vi "Vibration.vi"() -> ()   [LabVIEW 2012]
uses:
  <vilib>/Analysis/NI_AALPro.lvlib
panel:
  out "选项卡":T1(tab)
  in  "装置IP":string
  in  "?":bool
  in  "采样率(ksps)":T2(ring)=enum."105.468"
  in  "?":bool
  in  "?":bool
  in  "开始":bool
  in  "?":bool
  in  "设置装置网关":string
  in  "设置装置子网掩码":string
  in  "设置装置IP":string
  in  "?":bool
  in  "是否开启电流源":u8(knob)=1 scale=0.0..1.0
  in  "是否进行自校准":u8(knob) scale=0.0..1.0
  in  "?":bool
  in  "?":path
  in  "是否保存数据":u8(knob) scale=0.0..1.0
  in  "?":bool
  out "进度条":dbl(slide) scale=0.0..99.0
  out "字符串":string
  out "波形卡":enum32{"波形卡 1", "波形卡 2", "波形卡 3"}(tab)
  in  "AC/DC":bool
  in  "Y轴调整":dbl(knob)=5.0 min=0.0001 max=5.0 step=0.001 scale=0.0001..5.0
  out "?":dbl[][](graph)
  out "?":dbl[][](graph)
  in  "X轴调整":u32(knob)=50000 min=1000 max=50000 step=100 scale=1100.0..50000.0
  in  "通道1":bool=TRUE
  in  "通道2":bool=TRUE
  in  "通道3":bool=TRUE
  in  "通道4":bool=TRUE
  in  "灵敏度1(mv/g)":i32=1 min=1
  in  "灵敏度2(mv/g)":i32=1 min=1
  in  "灵敏度3(mv/g)":i32=1 min=1
  in  "灵敏度4(mv/g)":i32=1 min=1
  out "?":u16[](graph)
  out "转 \n速":u16(knob) scale=0.0..20000.0
  # "PageUp\nPageDown\n微调"
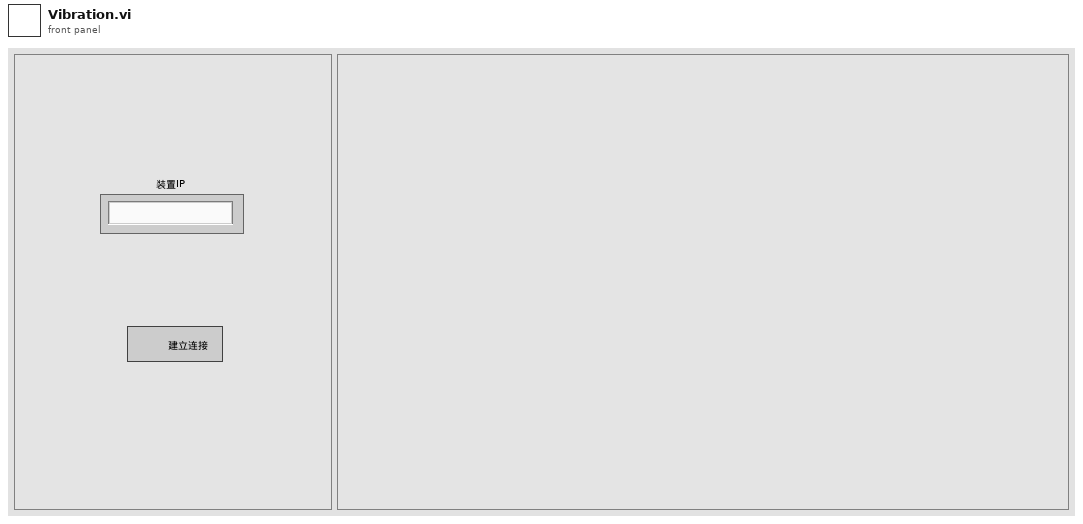
[diagram p1: front panel]
types:
  T1 = enum32{"选项卡 1", "选项卡 2", "选项卡 3", "选项卡 4", "选项卡 5", "选项卡 6", "选项卡 7"}
  T2 = enum16{"", "105.468", "52.734", "35.156", "26.367", "21.094", "17.578", "15.067", "13.184", "11.719", "10.545"}
  T3 = enum8{"Enabled", "Disabled", "Disabled and Grayed Out"}
  T4 = cluster{"refnum":refnum<file>, "refnum":refnum<file>, "refnum":refnum<file>, "refnum":refnum<file>, "refnum":refnum<file>, "SavePath":path, "SAVE?":bool, "connection ID":refnum<k5>}
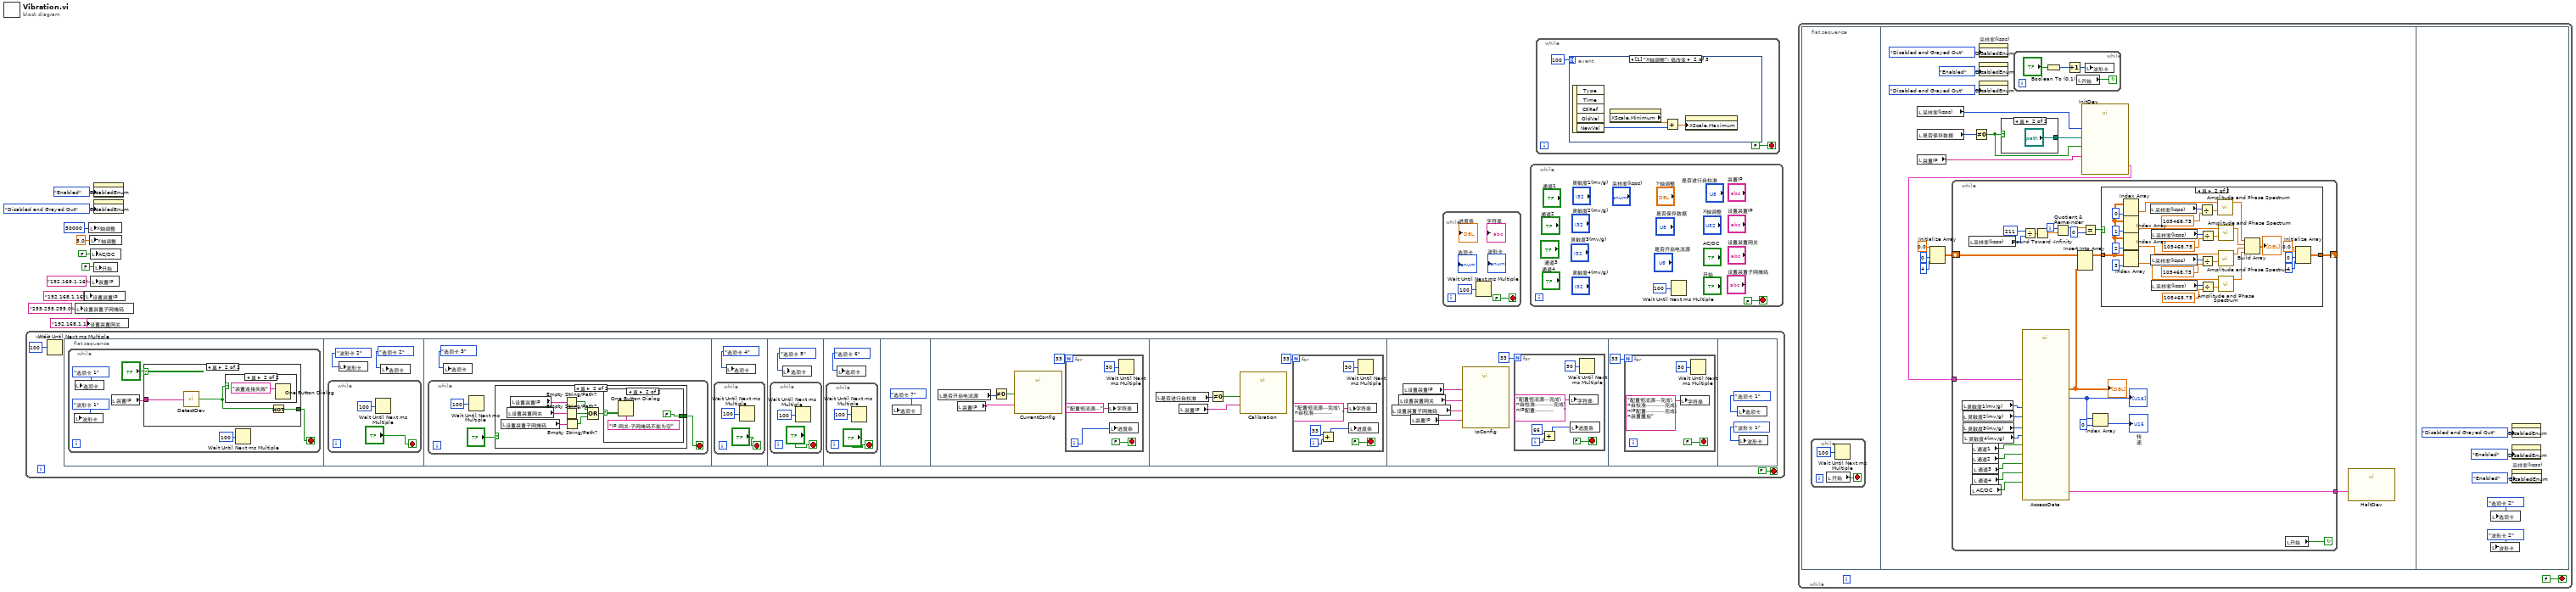
[diagram p0: block diagram]
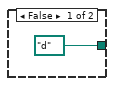
[diagram p3: hidden frame]
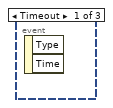
[diagram p4: hidden frame]
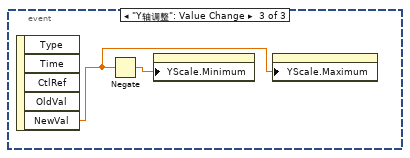
[diagram p5: hidden frame]
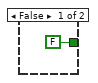
[diagram p6: hidden frame]
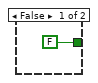
[diagram p8: hidden frame]
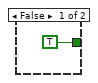
[diagram p9: hidden frame]
diagram:
  n1 = while {
    stop <- FALSE stop-if-true
    n2 = Wait Until Next ms Multiple(millisecond multiple=u32 100 ("毫秒倍数")) -> ()  [unwired: 1 out]
    n3 = flat-sequence {
      frame #0 {
        n4 = while {
          stop <- w17 stop-if-true
          n5 = local write "波形卡"(enum32{"波形卡 1", "波形卡 2", "波形卡 3"}."波形卡 1" ("波形卡")) -> ()
          n6 = local write "选项卡"(T1."选项卡 1" ("选项卡")) -> ()
          n7 = local read "装置IP"() -> (w13:string)
          n8 = case shown="真" "?" {
            tunnel: [FALSE w22] -> w17
            tunnel: w13 -> [_ w20]
            frame False {
            }
            frame True {
              n9 = call "DetectDev.vi"("IP."=w20) -> ("Fail"=w21:bool)
              n10 = case shown="真" w21 {
                frame False {
                }
                frame True {
                  n11 = One Button Dialog(message="装置连接失败" ("消息")) -> ()  [unwired: 1 in, 1 out]
                }
              }
              n12 = Not(x=w21) -> (.not. x?=w22:bool)
            }
          }
          n13 = Wait Until Next ms Multiple(millisecond multiple=u32 100 ("毫秒倍数")) -> ()  [unwired: 1 out]
        }
      }
      frame #1 {
        n14 = while {
          stop <- "?" stop-if-true
          n15 = Wait Until Next ms Multiple(millisecond multiple=u32 100 ("毫秒倍数")) -> ()  [unwired: 1 out]
        }
        n16 = local write "波形卡"(enum32{"波形卡 1", "波形卡 2", "波形卡 3"}."波形卡 2" ("波形卡")) -> ()
        n17 = local write "选项卡"(T1."选项卡 2" ("选项卡")) -> ()
      }
      frame #2 {
        n18 = while {
          stop <- w29 stop-if-true
          n19 = Wait Until Next ms Multiple(millisecond multiple=u32 100 ("毫秒倍数")) -> ()  [unwired: 1 out]
          n20 = case shown="真" "?" {
            tunnel: [FALSE w33] -> w29
            frame False {
            }
            frame True {
              n21 = local read "设置装置子网掩码"() -> (w40:string)
              n22 = local read "设置装置网关"() -> (w39:string)
              n23 = local read "设置装置IP"() -> (w38:string)
              n24 = Empty String/Path?(string/path=w38) -> (empty?=w35:bool)
              n25 = Empty String/Path?(string/path=w39) -> (empty?=w36:bool)
              n26 = Empty String/Path?(string/path=w40) -> (empty?=w37:bool)
              n27 = Compound Arithmetic op=OR(w35, w36, w37) -> (w34:bool)
              n28 = case shown="真" w34 {
                tunnel: [TRUE FALSE] -> w33
                frame False {
                }
                frame True {
                  n29 = One Button Dialog(message="IP,网关,子网掩码不能为空" ("消息")) -> ()  [unwired: 1 in, 1 out]
                }
              }
            }
          }
        }
        n30 = local write "选项卡"(T1."选项卡 3" ("选项卡")) -> ()
      }
      frame #3 {
        n31 = while {
          stop <- "?" stop-if-true
          n32 = Wait Until Next ms Multiple(millisecond multiple=u32 100 ("毫秒倍数")) -> ()  [unwired: 1 out]
        }
        n33 = local write "选项卡"(T1."选项卡 4" ("选项卡")) -> ()
      }
      frame #4 {
        n34 = while {
          stop <- "?" stop-if-true
          n35 = Wait Until Next ms Multiple(millisecond multiple=u32 100 ("毫秒倍数")) -> ()  [unwired: 1 out]
        }
        n36 = local write "选项卡"(T1."选项卡 5" ("选项卡")) -> ()
      }
      frame #5 {
        n37 = while {
          stop <- "?" stop-if-true
          n38 = Wait Until Next ms Multiple(millisecond multiple=u32 100 ("毫秒倍数")) -> ()  [unwired: 1 out]
        }
        n39 = local write "选项卡"(T1."选项卡 6" ("选项卡")) -> ()
      }
      frame #6 {
        n40 = local write "选项卡"(T1."选项卡 7" ("选项卡")) -> ()
      }
      frame #7 {
        n41 = local read "是否开启电流源"() -> (w55:u8)
        n42 = local read "装置IP"() -> (w54:string)
        n43 = Not Equal To 0?(x=w55) -> (x != 0?=w56:bool)
        n44 = call "CurrentConfig.vi"("Current"=w56, "IP"=w54) -> ()
        n45 = for {
          N: 33 -> [_]
          i -> [w58]
          stop <- FALSE stop-if-true
          n46 = local write "字符串"("配置恒流源..." ("字符串")) -> ()
          n47 = local write "进度条"(w58) -> ()
          n48 = Wait Until Next ms Multiple(millisecond multiple=u32 50 ("毫秒倍数")) -> ()  [unwired: 1 out]
        }
      }
      frame #8 {
        n49 = local read "是否进行自校准"() -> (w63:u8)
        n50 = local read "装置IP"() -> (w62:string)
        n51 = Not Equal To 0?(x=w63) -> (x != 0?=w64:bool)
        n52 = call "Calibration.vi"("Enable"=w64, "IP."=w62) -> ()
        n53 = for {
          N: 33 -> [_]
          i -> [w68]
          stop <- FALSE stop-if-true
          n54 = Add(x=33, y=w68) -> (x+y=w67:i32)
          n55 = local write "字符串"("配置恒流源...完成\n自校准...........      " ("字符串")) -> ()
          n56 = local write "进度条"(w67) -> ()
          n57 = Wait Until Next ms Multiple(millisecond multiple=u32 50 ("毫秒倍数")) -> ()  [unwired: 1 out]
        }
      }
      frame #9 {
        n58 = local read "设置装置子网掩码"() -> (w74:string)
        n59 = local read "设置装置网关"() -> (w73:string)
        n60 = local read "设置装置IP"() -> (w72:string)
        n61 = local read "装置IP"() -> (w75:string)
        n62 = call "IpConfig.vi"("Gateway"=w73, "SubnetMask"=w74, "IP"=w72, "CurrentIP"=w75) -> ()
        n63 = for {
          N: 33 -> [_]
          i -> [w79]
          stop <- FALSE stop-if-true
          n64 = Add(x=66, y=w79) -> (x+y=w78:i32)
          n65 = local write "字符串"("配置恒流源...完成\n自校准...........完成\nIP配置...........      " ("字符串")) -> ()
          n66 = local write "进度条"(w78) -> ()
          n67 = Wait Until Next ms Multiple(millisecond multiple=u32 50 ("毫秒倍数")) -> ()  [unwired: 1 out]
        }
      }
      frame #10 {
        n68 = for {
          N: 33 -> [_]
          stop <- FALSE stop-if-true
          n69 = local write "字符串"("配置恒流源...完成\n自校准...........完成\nIP配置...........完成\n装置重启" ("字符串")) -> ()
          n70 = Wait Until Next ms Multiple(millisecond multiple=u32 50 ("毫秒倍数")) -> ()  [unwired: 1 out]
        }
      }
      frame #11 {
        n71 = local write "选项卡"(T1."选项卡 1" ("选项卡")) -> ()
        n72 = local write "波形卡"(enum32{"波形卡 1", "波形卡 2", "波形卡 3"}."波形卡 1" ("波形卡")) -> ()
      }
    }
  }
  n73 = local write "设置装置子网掩码"("255.255.255.0" ("新子网掩码")) -> ()
  n74 = local write "设置装置网关"("192.168.1.1" ("新网关")) -> ()
  n75 = local write "设置装置IP"("192.168.1.16" ("新装置IP")) -> ()
  n76 = local write "X轴调整"(u16 50000 ("X轴调整")) -> ()
  n77 = local write "Y轴调整"(5.0 ("Y轴调整")) -> ()
  n78 = local write "AC/DC"(FALSE ("AC/DC")) -> ()
  n79 = local write "装置IP"("192.168.1.16" ("装置IP")) -> ()
  n80 = property class="Bool"("DisabledEnum"=T3."Enabled" ("禁用")) -> ()  [unwired: 2 in, 2 out]
  n81 = property class="Bool (严格)"("DisabledEnum"=T3."Disabled and Grayed Out" ("禁用")) -> ()  [unwired: 2 in, 2 out]
  n82 = local write "开始"(FALSE ("开始")) -> ()
  n83 = while {
    stop <- FALSE stop-if-true
    n84 = Wait Until Next ms Multiple(millisecond multiple=u32 100 ("毫秒倍数")) -> ()  [unwired: 1 out]
  }
  n85 = while {
    stop <- FALSE stop-if-true
    n86 = Wait Until Next ms Multiple(millisecond multiple=u32 100 ("毫秒倍数")) -> ()  [unwired: 1 out]
  }
  n87 = while {
    stop <- FALSE stop-if-true
    n88 = event shown="[1] \"X轴调整\": 值改变" {
      selector: _ -> [_ _ _]
      dyn-events: _ -> [_ _ _]
      timeout: 100 -> [_ _ _]
      event Timeout {
        n89 = event-data() -> ()  [unwired: 1 in, 2 out]
      }
      event "X轴调整": Value Change {
        n90 = event-data() -> ("NewVal"=w97:u32)  [unwired: 1 in, 4 out]
        n91 = property class="WFChart (严格)"() -> ("XScale.Minimum"=w96:dbl)  [unwired: 2 in, 2 out]
        n92 = Add(x=w96, y=w97) -> (x+y=w95:dbl)
        n93 = property class="WFChart (严格)"("XScale.Maximum"=w95) -> ()  [unwired: 2 in, 2 out]
      }
      event "Y轴调整": Value Change {
        n94 = event-data() -> ("NewVal"=w98:dbl)  [unwired: 1 in, 4 out]
        n95 = Negate(x=w98) -> (-x=w99:dbl)
        n96 = property class="WFChart (严格)"("YScale.Minimum"=w99) -> ()  [unwired: 2 in, 2 out]
        n97 = property class="WFChart (严格)"("YScale.Maximum"=w98) -> ()  [unwired: 2 in, 2 out]
      }
    }
  }
  n98 = while {
    stop <- FALSE stop-if-true
    n99 = flat-sequence {
      frame #0 {
        n100 = while {
          stop <- w101 stop-if-true
          n101 = local read "开始"() -> (w101:bool)
          n102 = Wait Until Next ms Multiple(millisecond multiple=u32 100 ("毫秒倍数")) -> ()  [unwired: 1 out]
        }
      }
      frame #1 {
        n103 = local read "采样率(ksps)"() -> (w104:T2)
        n104 = local read "是否保存数据"() -> (w116:u8)
        n105 = local read "装置IP"() -> (w111:string)
        n106 = Initialize Array(0.0 ("元素"), 0 ("维数大小"), 4 ("维数大小")) -> (w105:dbl[][])
        n107 = Not Equal To 0?(x=w116) -> (x != 0?=w112:bool)
        n108 = property on="采样率(ksps)" class="Enum (严格)"("DisabledEnum"=T3."Disabled and Grayed Out" ("禁用")) -> ()  [unwired: 2 in, 2 out]
        n109 = property class="Bool (严格)"("DisabledEnum"=T3."Enabled" ("禁用")) -> ()  [unwired: 2 in, 2 out]
        n110 = property class="Bool"("DisabledEnum"=T3."Disabled and Grayed Out" ("禁用")) -> ()  [unwired: 2 in, 2 out]
        n111 = case shown="真" w112 {
          tunnel: [path "d:/" ("路径（使用对话框）") "?"] -> w113
          frame False {
          }
          frame True {
          }
        }
        n112 = while {
          stop <- w175 continue-if-true
          n113 = Boolean To (0,1)(Boolean="?") -> (0, 1=w178:i16)
          n114 = Increment(x=w178) -> (x+1=w176:i16)
          n115 = local read "开始"() -> (w175:bool)
          n116 = local write "波形卡"(w176) -> ()
        }
        n117 = call "InitDev.vi"("SAVE?"=w112, "IP地址"=w111, "SampleRate"=w104, "SavePath"=w113) -> ("输出簇"=w110:T4)
        n118 = while {
          tunnel: w110 -> [w140]
          tunnel: [w139] -> w109
          shift-right: [w135] -> _
          shift-left: w105 -> [w137]
          i -> [w132]
          stop <- w141 continue-if-true
          n119 = local read "灵敏度1(mv/g)"() -> (w125:i32)
          n120 = local read "灵敏度2(mv/g)"() -> (w124:i32)
          n121 = local read "灵敏度3(mv/g)"() -> (w123:i32)
          n122 = local read "灵敏度4(mv/g)"() -> (w122:i32)
          n123 = local read "采样率(ksps)"() -> (w129:T2)
          n124 = local read "AC/DC"() -> (w117:bool)
          n125 = local read "通道1"() -> (w121:bool)
          n126 = local read "通道2"() -> (w120:bool)
          n127 = local read "通道3"() -> (w119:bool)
          n128 = local read "通道4"() -> (w118:bool)
          n129 = call "AccessData.vi"("Sensitivity1"=w125, "CH1Enable"=w121, "Sensitivity2"=w124, "CH2Enable"=w120, "Sensitivity3"=w123, "CH3Enable"=w119, "Sensitivity4"=w122, "CH4Enable"=w118, "输入簇"=w140, "RmOffset"=w117) -> ("VibrationWave"=w126:dbl[][], "Speed"=w138:u16[], "输出簇"=w139:T4)  [unwired: 2 in, 1 out]
          "?" <- w126
          "?" <- w138
          n130 = Divide(x=u8 211, y=w129) -> (x/y=w130:dbl)
          n131 = Round Toward -Infinity(1:w130) -> (0:w128:dbl)
          n132 = Quotient & Remainder(x=w132, y=w128) -> (x-y*floor(x/y)=w134:dbl)  [unwired: 1 out]
          n133 = Insert Into Array(array=w137, new element=w126) -> (w136:dbl[][])  [unwired: 2 in]
          n134 = Equal?(x=w134, y=0) -> (x = y?=w127:bool)
          n135 = Index Array(array=w138, index=0 ("索引")) -> (element=→"转 \n速":u16)
          n136 = case shown="真" w127 {
            tunnel: w136 -> [w144 w151]
            tunnel: [w144 w147] -> w135
            frame False {
            }
            frame True {
              n137 = Index Array(array=w151, index (col)=0 ("禁用的索引 (列)")) -> (element=w153:dbl[])  [unwired: 1 in]
              n138 = Index Array(array=w151, index (col)=1 ("禁用的索引 (列)")) -> (element=w160:dbl[])  [unwired: 1 in]
              n139 = Index Array(array=w151, index (col)=2 ("禁用的索引 (列)")) -> (element=w159:dbl[])  [unwired: 1 in]
              n140 = Index Array(array=w151, index (col)=3 ("禁用的索引 (列)")) -> (element=w158:dbl[])  [unwired: 1 in]
              n141 = local read "采样率(ksps)"() -> (w170:T2)
              n142 = local read "采样率(ksps)"() -> (w164:T2)
              n143 = local read "采样率(ksps)"() -> (w167:T2)
              n144 = local read "采样率(ksps)"() -> (w161:T2)
              n145 = Divide(x=w170, y=105468.75 ("dt")) -> (x/y=w145:dbl)
              n146 = Divide(x=w164, y=105468.75 ("dt")) -> (x/y=w165:dbl)
              n147 = Divide(x=w167, y=105468.75 ("dt")) -> (x/y=w168:dbl)
              n148 = Divide(x=w161, y=105468.75 ("dt")) -> (x/y=w162:dbl)
              n149 = call <vilib>:"Amplitude and Phase Spectrum.vi"("dt"=w145, "Signal (V)"=w153) -> ("Amp Spectrum Mag (Vrms)"=w157:dbl[])  [unwired: 1 in, 2 out]
              n150 = call <vilib>:"Amplitude and Phase Spectrum.vi"("dt"=w165, "Signal (V)"=w159) -> ("Amp Spectrum Mag (Vrms)"=w154:dbl[])  [unwired: 1 in, 2 out]
              n151 = call <vilib>:"Amplitude and Phase Spectrum.vi"("dt"=w168, "Signal (V)"=w160) -> ("Amp Spectrum Mag (Vrms)"=w156:dbl[])  [unwired: 1 in, 2 out]
              n152 = call <vilib>:"Amplitude and Phase Spectrum.vi"("dt"=w162, "Signal (V)"=w158) -> ("Amp Spectrum Mag (Vrms)"=w155:dbl[])  [unwired: 1 in, 2 out]
              n153 = Build Array(w157, w156, w154, w155) -> (→"?":dbl[][])
              n154 = Initialize Array(0.0 ("元素"), 0 ("维数大小"), 4 ("维数大小")) -> (w147:dbl[][])
            }
          }
          n155 = local read "开始"() -> (w141:bool)
        }
        n156 = call "HaltDev.vi"("输入簇"=w109) -> ()
      }
      frame #2 {
        n157 = local write "波形卡"(enum32{"波形卡 1", "波形卡 2", "波形卡 3"}."波形卡 2" ("波形卡")) -> ()
        n158 = local write "选项卡"(T1."选项卡 2" ("选项卡")) -> ()
        n159 = property class="Bool (严格)"("DisabledEnum"=T3."Disabled and Grayed Out" ("禁用")) -> ()  [unwired: 2 in, 2 out]
        n160 = property class="Bool"("DisabledEnum"=T3."Enabled" ("禁用")) -> ()  [unwired: 2 in, 2 out]
        n161 = property on="采样率(ksps)" class="Enum (严格)"("DisabledEnum"=T3."Enabled" ("禁用")) -> ()  [unwired: 2 in, 2 out]
      }
    }
  }
